vi "VI Tree.vi"   [LabVIEW 2015, in "ZhiYuan ZDS Series for TCP.lvlib"]
doc: "This is the instrument driver for the ZDS 2000, 4000 Series oscilloscopes. The VI Tree displays all the user-callable VIs of the instrument driver in an organized table."
uses:
  ZhiYuan ZDS Series for TCP.lvlib
  Data/Read Waveform (Single).vi
  Configure/Math/Configure Math (Base).vi
  Configure/Trigger/Configure Trigger (Edge).vi
panel:
  # "(c) 2012 National Instruments.  ALL RIGHTS RESERVED."
  # "SEE DIAGRAM\nFOR VI TREE."
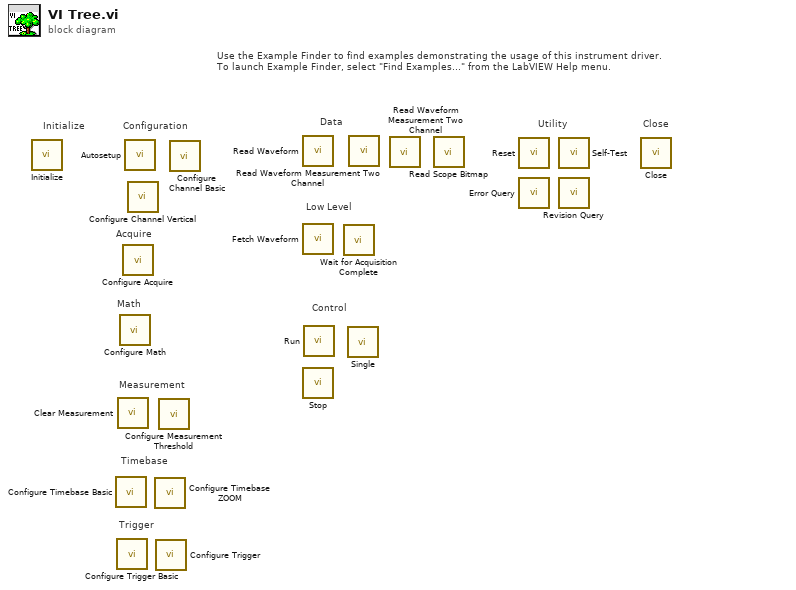
[diagram p0: block diagram]
diagram:
  # "Control"
  # "Trigger"
  # "Timebase"
  # "Measurement"
  # "Math"
  # "Acquire"
  # "Low Level"
  # "Use the Example Finder to find examples demonstrating the usage of this instrument driver.\nTo launch Example Finder, select \"Find Examples...\" from the LabVIEW Help menu."
  # "Configuration"
  # "Utility"
  # "Data"
  # "Close"
  # "Initialize"
  n1 = call "Initialize.vi"() -> ()  [unwired: 10 in, 2 out]
  n2 = call "Configure Timebase Basic.vi"() -> ()  [unwired: 14 in, 2 out]
  n3 = call "Configure Trigger Basic.vi"() -> ()  [unwired: 10 in, 2 out]
  n4 = call "Clear Measurement.vi"() -> ()  [unwired: 10 in, 2 out]
  n5 = call-poly "Configure Math.vi"() -> ()  [unwired: 14 in, 2 out]
  n6 = call "Configure Acquire.vi"() -> ()  [unwired: 10 in, 2 out]
  n7 = call "Autosetup.vi"() -> ()  [unwired: 10 in, 2 out]
  n8 = call "Configure Channel Vertical.vi"() -> ()  [unwired: 10 in, 2 out]
  n9 = call "Configure Timebase ZOOM.vi"() -> ()  [unwired: 10 in, 2 out]
  n10 = call-poly "Configure Trigger.vi"() -> ()  [unwired: 14 in, 2 out]
  n11 = call "Configure Measurement Threshold.vi"() -> ()  [unwired: 10 in, 2 out]
  n12 = call "Configure Channel Basic.vi"() -> ()  [unwired: 14 in, 2 out]
  n13 = call-poly "Read Waveform.vi"() -> ()  [unwired: 9 in, 3 out]
  n14 = call "Fetch Waveform.vi"() -> ()  [unwired: 9 in, 3 out]
  n15 = call "Stop.vi"() -> ()  [unwired: 10 in, 2 out]
  n16 = call "Run.vi"() -> ()  [unwired: 10 in, 2 out]
  n17 = call "Wait for Acquisition Complete.vi"() -> ()  [unwired: 10 in, 2 out]
  n18 = call "Single.vi"() -> ()  [unwired: 10 in, 2 out]
  n19 = call "Read Waveform Measurement Two Channel.vi"() -> ()  [unwired: 9 in, 3 out]
  n20 = call "Read Waveform Measurement Two Channel.vi"() -> ()  [unwired: 9 in, 3 out]
  n21 = call "Read Scope Bitmap.vi"() -> ()  [unwired: 9 in, 3 out]
  n22 = call "Reset.vi"() -> ()  [unwired: 10 in, 2 out]
  n23 = call "Error Query.vi"() -> ()  [unwired: 8 in, 4 out]
  n24 = call "Self-Test.vi"() -> ()  [unwired: 8 in, 4 out]
  n25 = call "Revision Query.vi"() -> ()  [unwired: 8 in, 4 out]
  n26 = call "Close.vi"() -> ()  [unwired: 11 in, 1 out]
